vi "邮件通知密码.vi"(10 "收件人Email":string, 11 "PC总客户端.i":refnum<class "PC总客户端.lvclass">) -> ()   [LabVIEW 2013, in "个人剂量仪-云服务器.lvclass"]
uses:
  <vilib>/Utility/config.llb/Read Key (String).vi
  <vilib>/smtpClient/Set Message Text.vi
  <vilib>/smtpClient/LabVIEWSMTPClient.lvlib
  <vilib>/Utility/config.llb/NI_LVConfig.lvlib
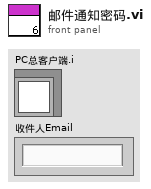
[diagram p1: front panel]
types:
  T1 = cluster{"登录名":string, "密码":string, "企业名称":string, "邮箱":string, "电话":string}
  T2 = typedef "NI_LVConfig.lvlib/Config Data RefNum.ctl" = refnum<k1>
  T3 = typedef "LabVIEWSMTPClient.lvlib/SmtpClientHandle.ctl" = refnum<k1>
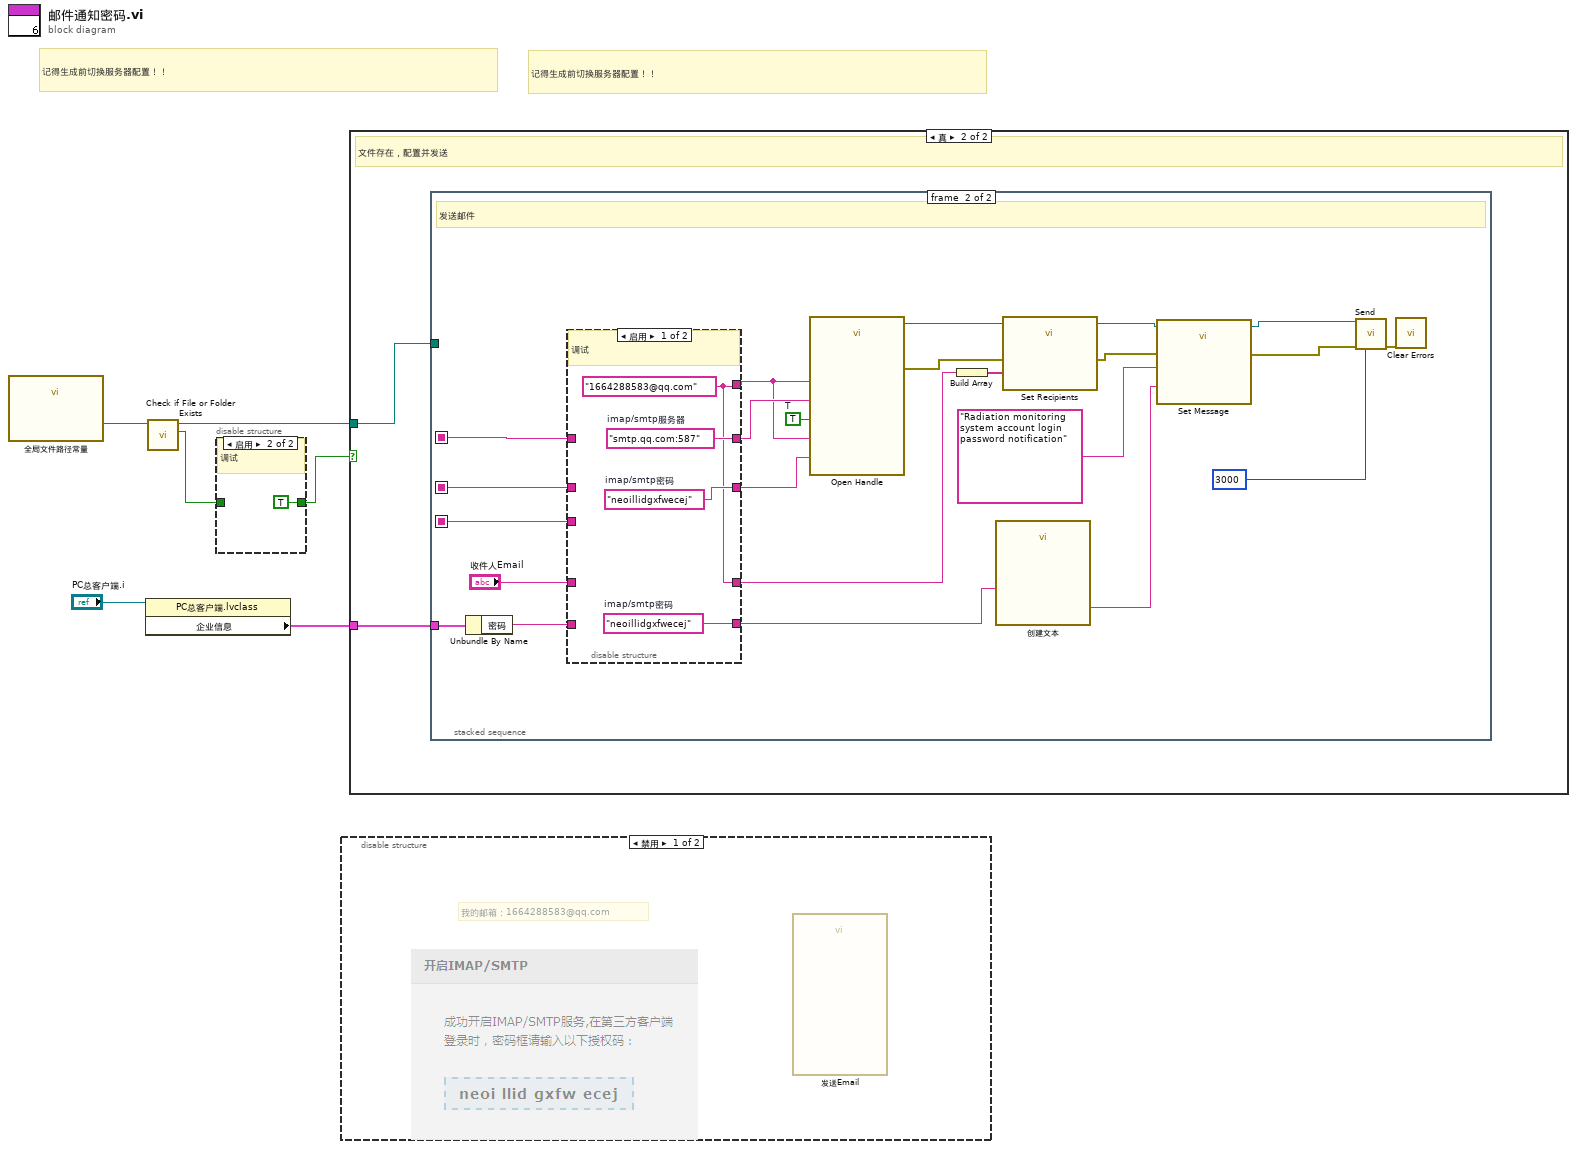
[diagram p0: block diagram]
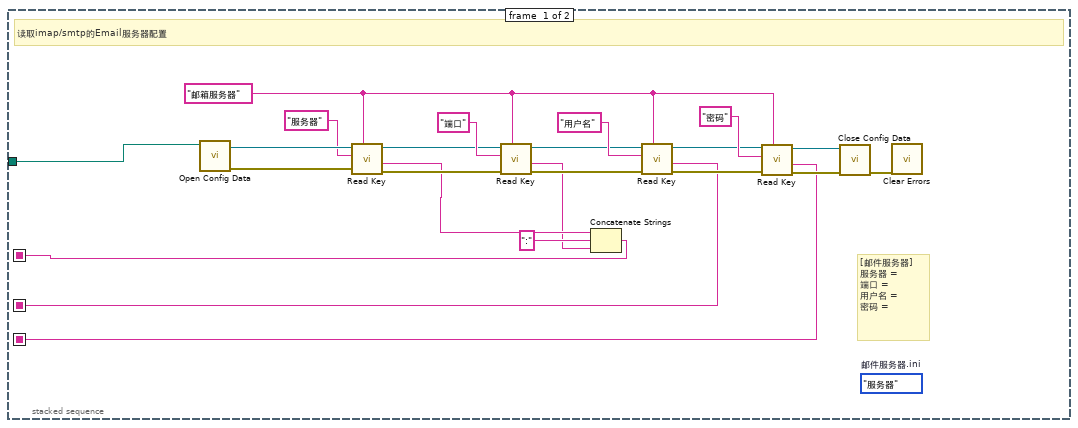
[diagram p4: hidden frame]
diagram:
  # "记得生成前切换服务器配置！！"
  # "记得生成前切换服务器配置！！"
  n1 = call "全局文件路径常量.vi"() -> ("Email服务器配置"=w6:path)  [unwired: 9 in, 2 out]
  n2 = property class="PC总客户端.lvclass"(reference="PC总客户端.i") -> ("企业信息"=w4:T1)  [unwired: 1 in, 2 out]
  n3 = call <vilib>:"Check if File or Folder Exists.vi"("path"=w6) -> ("file or folder exists?"=w2:bool, "dup path"=w3:path)  [unwired: 8 in, 1 out]
  n4 = disable-structure shown="启用" {
    disable-tunnel: w2 -> [w7 _]
    disable-tunnel: [w7 TRUE ("file or folder exists?")] -> w1
    frame Disabled {
      # "产品"
    }
    frame Enabled {
      # "调试"
    }
  }
  n5 = disable-structure shown="禁用" {
    frame Disabled {
      # "我的邮箱：1664288583@qq.com"
      n6 = call "发送Email"() -> ()  [unwired: 11 in, 1 out]
    }
    frame Enabled {
    }
  }
  n7 = case shown="真" w1 {
    tunnel: w4 -> [_ w9]
    tunnel: w3 -> [_ w10]
    frame False {
      # "配置文件不存在，不发送"
    }
    frame True {
      # "文件存在，配置并发送"
      n8 = stacked-sequence {
        seq-local: [w12 _] -> [_ w50]
        seq-local: [w17 _] -> [_ w47]
        seq-local: [w16 _] -> [_ w46]
        tunnel: w10 -> [w33 _]
        tunnel: w9 -> [_ w44]
        frame #0 {
          (unwired) enum16{"服务器", "端口", "用户名", "密码"}."服务器"  # 邮件服务器.ini
          w30 = "邮箱服务器" ("section")
          # "[邮件服务器]\n服务器 =\n端口 =\n用户名 =\n密码 ="
          # "读取imap/smtp的Email服务器配置"
          n9 = call <vilib>:"Open Config Data.vi"("configuration file path"=w33) -> ("error out"=w22:errorcluster, "refnum"=w32:T2)  [unwired: 8 in, 1 out]
          n10 = call-poly <vilib>:"Read Key.vi"("section"=w30, "error in (no error)"=w22, "key"="服务器", "refnum"=w32) -> ("error out"=w21:errorcluster, "value"=w14:string, "refnum out"=w26:T2)  [unwired: 4 in, 1 out]
          n11 = call-poly <vilib>:"Read Key.vi"("section"=w30, "error in (no error)"=w21, "key"="端口", "refnum"=w26) -> ("error out"=w20:errorcluster, "value"=w13:string, "refnum out"=w25:T2)  [unwired: 4 in, 1 out]
          n12 = Concatenate Strings(w14, ":" ("字符串"), w13) -> (w12:string)
          n13 = call-poly <vilib>:"Read Key.vi"("section"=w30, "error in (no error)"=w20, "key"="用户名", "refnum"=w25) -> ("error out"=w19:errorcluster, "value"=w17:string, "refnum out"=w24:T2)  [unwired: 4 in, 1 out]
          n14 = call-poly <vilib>:"Read Key.vi"("section"=w30, "error in (no error)"=w19, "key"="密码", "refnum"=w24) -> ("error out"=w18:errorcluster, "value"=w16:string, "refnum out"=w23:T2)  [unwired: 4 in, 1 out]
          n15 = call <vilib>:"Close Config Data.vi"("error in (no error)"=w18, "refnum"=w23) -> ("error out"=w11:errorcluster)  [unwired: 8 in, 1 out]
          n16 = call <vilib>:"Clear Errors.vi"("error in (no error)"=w11) -> ()  [unwired: 6 in, 1 out]
        }
        frame #1 {
          w55 = TRUE  # T
          # "发送邮件"
          n17 = Unbundle By Name(w44) -> ("密码"=w42:string)
          n18 = disable-structure shown="启用" {
            disable-tunnel: [w60 w65] -> w56
            disable-tunnel: w50 -> [_ w65]
            disable-tunnel: [w57 w63] -> w49
            disable-tunnel: [w59 w64] -> w48
            disable-tunnel: w47 -> [_ w63]
            disable-tunnel: w46 -> [_ w64]
            disable-tunnel: w42 -> [_ w62]
            disable-tunnel: [w58 w62] -> w41
            disable-tunnel: [w57 w61] -> w40
            disable-tunnel: "收件人Email" -> [_ w61]
            frame Enabled {
              w58 = "neoillidgxfwecej"  # imap/smtp密码
              w57 = "1664288583@qq.com" ("from")
              w59 = "neoillidgxfwecej"  # imap/smtp密码
              w60 = "smtp.qq.com:587"  # imap/smtp服务器
              # "调试"
            }
            frame Disabled {
              # "产品"
            }
          }
          n19 = call <vilib>:"Open Handle.vi"("server address"=w56, "from"=w49, "username"=w49, "password"=w48, "use TLS (false)"=w55) -> ("handle out"=w54:T3, "error out"=w37:errorcluster)  [unwired: 9 in]
          n20 = Build Array(w40) -> (w45:string[])
          n21 = call "创建文本"("密码"=w41) -> ("Result"=w43:string)  [unwired: 13 in, 1 out]
          n22 = call <vilib>:"Set Recipients.vi"("handle in"=w54, "to"=w45, "error in (no error)"=w37) -> ("handle out"=w53:T3, "error out"=w36:errorcluster)  [unwired: 11 in]
          n23 = call-poly <vilib>:"Set Message.vi"("handle in"=w53, "subject"="Radiation monitoring system account login password notification" ("from"), "plain text message"=w43, "error in (no error)"=w36) -> ("handle out"=w52:T3, "error out"=w35:errorcluster)  [unwired: 10 in]
          n24 = call <vilib>:"Send.vi"("handle in"=w52, "error in (no error)"=w35, "timeout in ms (10000)"=3000) -> ("error out"=w38:errorcluster)  [unwired: 10 in, 2 out]
          n25 = call <vilib>:"Clear Errors.vi"("error in (no error)"=w38) -> ()  [unwired: 6 in, 1 out]
        }
      }
    }
  }
